vi "SendActorCoreMsg.vi"(8 "error in (no error)":errorcluster, 9 "Data":variant, 10 "Msg":T1, 11 "DAQ_Module in":refnum<class "DAQ_Module.lvclass">) -> (0 "error out":errorcluster, 3 "DAQ_Module out":refnum<class "DAQ_Module.lvclass">)   [LabVIEW 2025]
uses:
  DAQ_Module.lvclass
  Msg.ctl
  Msg&Data.ctl
  DAQ_Module.lvclass/DAQ_Module.ctl
  C:/Program Files (x86)/National Instruments/LabVIEW 2025/vi.lib/ActorFramework/Actor/Actor.lvclass
  D:/Hardware/DAQ/DAQ_Module/DAQ_Module/DAQ_Module/DAQ_Module.lvclass
  D:/Hardware/Module/Module/Module_Interface/Module_Interface.lvclass
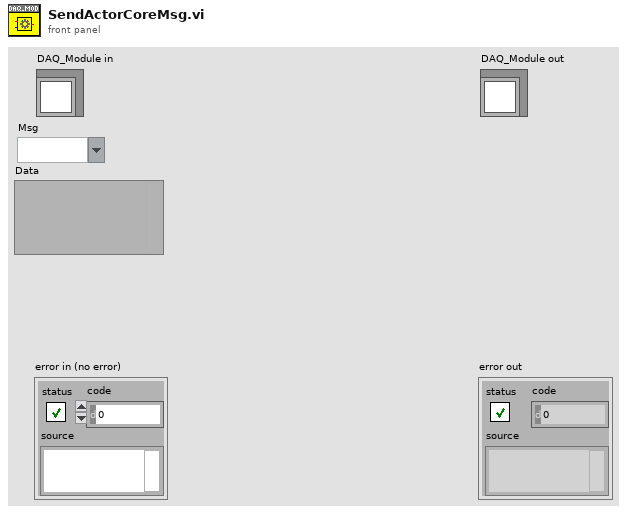
[diagram p1: front panel]
types:
  T1 = typedef "Msg.ctl" = string
  T2 = typedef "Msg&Data.ctl" = cluster{"Msg":T1, "Data":variant}
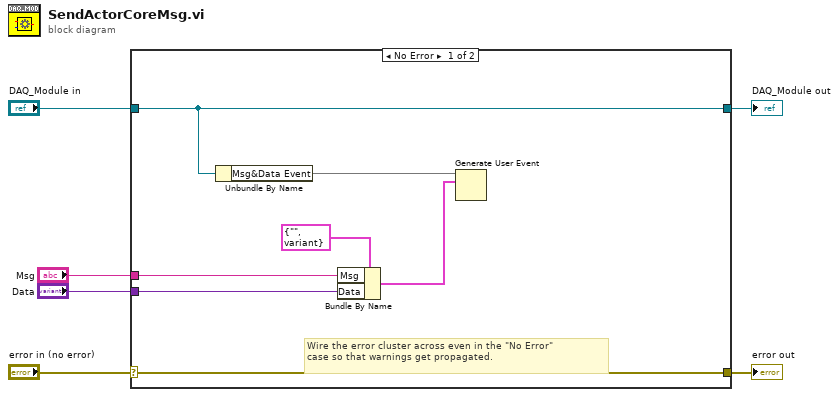
[diagram p0: block diagram]
diagram:
  n1 = case shown="No Error" "error in (no error)" {
    selector: "error in (no error)" -> [w13 w15]
    tunnel: [w13 w15] -> w5
    tunnel: [w9 w14] -> w3
    tunnel: "DAQ_Module in" -> [w9 w14]
    tunnel: "Data" -> [w8 _]
    tunnel: "Msg" -> [w7 _]
    frame No Error {
      # "Wire the error cluster across even in the \"No Error\"\ncase so that warnings get propagated."
      n2 = Unbundle By Name(w9) -> ("Msg&Data Event"=w12)
      n3 = Bundle By Name(cluster=T2 {"Msg"="", "Data"=variant} ("Msg&Data"), "Msg"=w7, "Data"=w8) -> (w10:T2)
      n4 = Generate User Event(user event=w12, event data cluster=w10) -> ()  [unwired: 2 in, 2 out]
    }
    frame Error {
    }
  }
  "error out" <- w5
  "DAQ_Module out" <- w3
